vi "Global-Settings.vi"() -> ()   [LabVIEW 2017]
uses:
  TypeDefs/Global-Settings-TD.ctl
panel:
  in  "Global Settings":T1
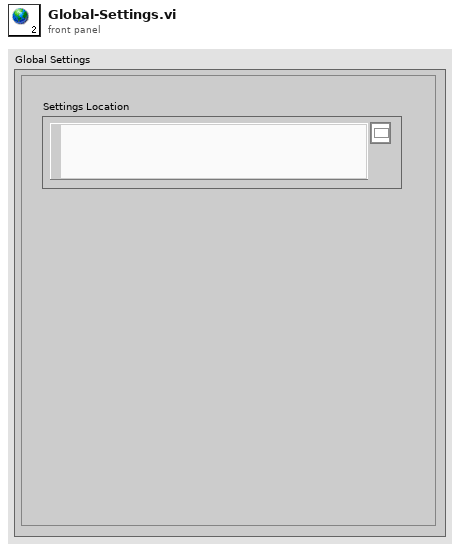
[diagram p1: front panel]
types:
  T1 = typedef "Global-Settings-TD.ctl" = cluster{"Settings Location":path}
diagram:
